vi "GV_GetSelProperties.vi"(8 "error in (no error)":errorcluster, 11 "Gviewer in":refnum<class "Gviewer.lvclass">) -> (0 "error out":errorcluster, 1 "Bool_id":bool[](array[boolean]), 2 "AllSelProps":T1[](array[typedef]) {"TAGprop"."TagFunc" format="%08x"; "TAGprop"."RangeL" format="%.2f"; "TAGprop"."RangeH" format="%.2f"}, 3 "Gviewer out":refnum<class "Gviewer.lvclass">)   [LabVIEW 2020, in "Sgraph_lib_V1.lvlib" / "Gviewer.lvclass"]
doc: "Get the TAG properties of the TAG selection list"
uses:
  Gviewer.lvclass
  DBAL/controls/DBAL_TAGpropEdit.ctl
  Common/controls/typedef_com_TagProp.ctl
  Gviewer.lvclass/Gviewer.ctl
  Builds/Sgraph_lib_V1.lvlib
  DBAL/DBAL.lvclass
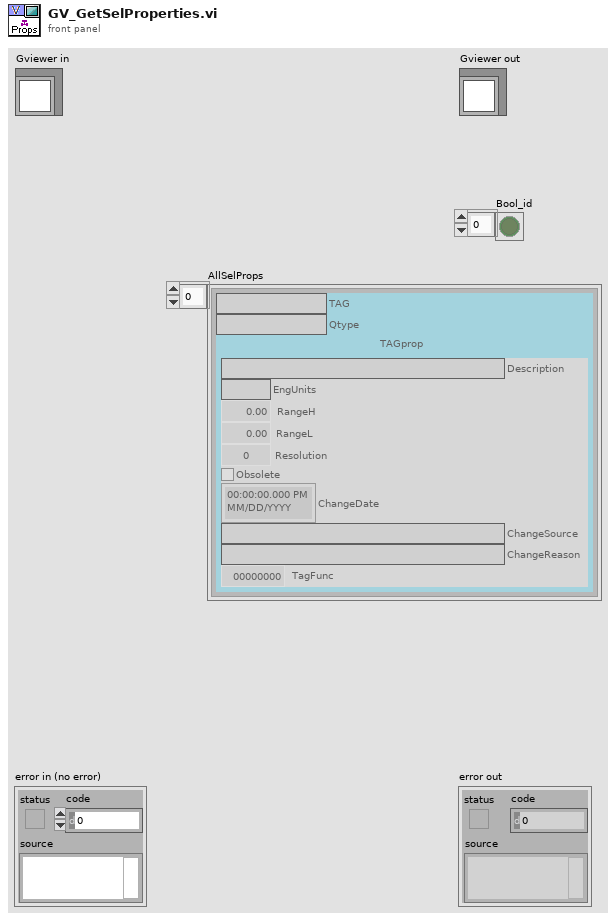
[diagram p1: front panel]
types:
  T1 = typedef "Sgraph_lib_V1.lvlib/DBAL.lvclass/DBAL_TAGpropEdit.ctl" = cluster{"TAG":string, "Qtype":string, "TAGprop":T2}
  T2 = typedef "Sgraph_lib_V1.lvlib/typedef_com_TagProp.ctl" = cluster{"Description":string, "EngUnits":string, "RangeH":dbl, "RangeL":dbl, "Resolution":i32, "Obsolete":bool, "ChangeDate":timestamp, "ChangeSource":string, "ChangeReason":string, "TagFunc":u32}
  T3 = typedef "Sgraph_lib_V1.lvlib/DBAL.lvclass/DBAL_TAGprops.ctl" = T1[]
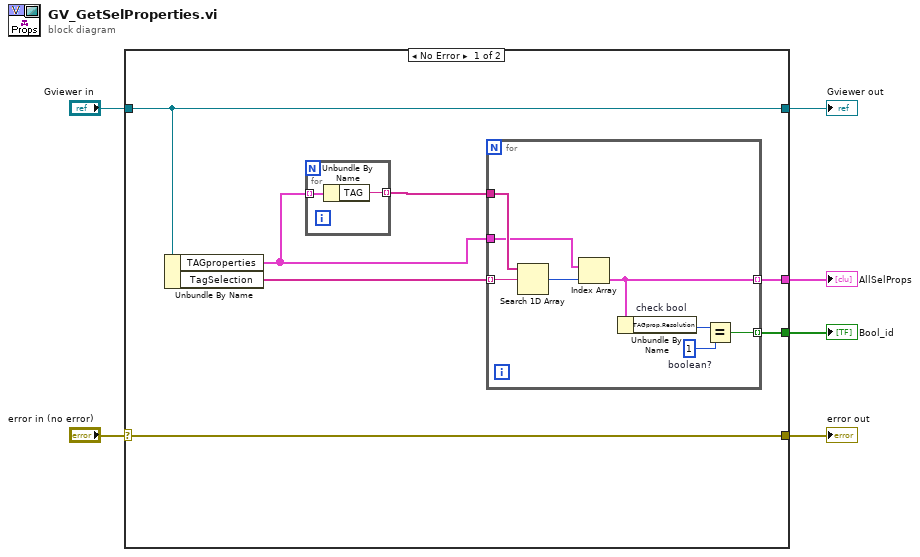
[diagram p0: block diagram]
diagram:
  n1 = case shown="No Error" "error in (no error)" {
    selector: "error in (no error)" -> [w13 w25]
    tunnel: [w13 w25] -> w5
    tunnel: [w10 w24] -> w3
    tunnel: "Gviewer in" -> [w10 w24]
    tunnel: [w8 _] -> w2
    tunnel: [w7 _] -> w1
    frame No Error {
      n2 = Unbundle By Name(w10) -> ("TAGproperties"=w9:T3, "TagSelection"=w12:string[])
      n3 = for {
        tunnel: w9 -> [w15] mode=indexing
        tunnel: [w14] -> w11 mode=indexing
        n4 = Unbundle By Name(w15) -> ("TAG"=w14:string)
      }
      n5 = for {
        tunnel: w12 -> [w21] mode=indexing
        tunnel: w11 -> [w20]
        tunnel: w9 -> [w19]
        tunnel: [w17] -> w7 mode=indexing
        tunnel: [w16] -> w8 mode=indexing
        w22 = 1  # boolean?
        n6 = Search 1D Array(1D array=w20, element=w21) -> (index of element=w18:i32)  [unwired: 1 in]
        n7 = Index Array(array=w19, index=w18) -> (element=w17:T1)
        n8 = Unbundle By Name "check bool"(w17) -> ("TAGprop.Resolution"=w23:i32)
        n9 = Equal?(x=w23, y=w22) -> (x = y?=w16:bool)
      }
    }
    frame Error {
    }
  }
  "error out" <- w5
  "Gviewer out" <- w3
  "Bool_id" <- w2
  "AllSelProps" <- w1
